vi "VTI_Split_Cluster.vi"(0 "VTI":T2={"Temperatur (K)"=0.0, "Setpoint (K)"=0.0, "Rate (K/min)"=3.4572, "Heater (%)"=0.0, "NV (%)"=0.0, "Heater Manual"=FALSE, "NV Manual"=FALSE, "Go to Set"=FALSE, "Pressure"=0.0, "Heater SP"=0.0, "Valid?"=FALSE, "Set Heater SP"=FALSE, "Set NV SP"=FALSE, "Heater (%) Display"=3.4572, "NV (%) Display"=3.4572, "NV Setpoint"=0.0, "Change Heater Status"=FALSE, "Change NV Status"=FALSE, "Sample 3"=0.0, "Sample 2"=0.0, "Sweep-State"=FALSE, "Set Auto PID"=FALSE, "Auto PID"=FALSE, "Stopp"=FALSE, "Setpoint-Sweep"=0.0} {"NV (%) Display" format="%4_5f"; "Heater (%) Display" format="%4_5f"; "Pressure" format="%#4_5f"; "NV (%)" scale=0.0..100.0; "Heater (%)" scale=0.0..100.0; "Rate (K/min)" format="%#4_5f"; "Setpoint (K)" format="%6_5f"}) -> (1 "VTI Status":T3={"Temperatur (K)"=70.6986, "Heater (%)"=0.0017142857142857142, "NV (%)"=0.0, "Heater Manual"=TRUE, "NV Manual"=TRUE, "Pressure"=1.0208606, "Valid?"=FALSE, "Heater (%) Display"=0.0, "NV (%) Display"=0.0, "Sample 2"=70.6986, "Sample 3"=70.6986, "Auto PID"=TRUE, "Sweep-Status"=TRUE, "Setpoint-Sweep"=70.6986} {"Heater (%)" scale=0.0..100.0; "NV (%)" scale=0.0..100.0}, 2 "VTI Control":T1)   [LabVIEW 2016]
uses:
  S16/VTI-status.ctl
  S16/VTI-cluster.ctl
  S16/VTI-control.ctl
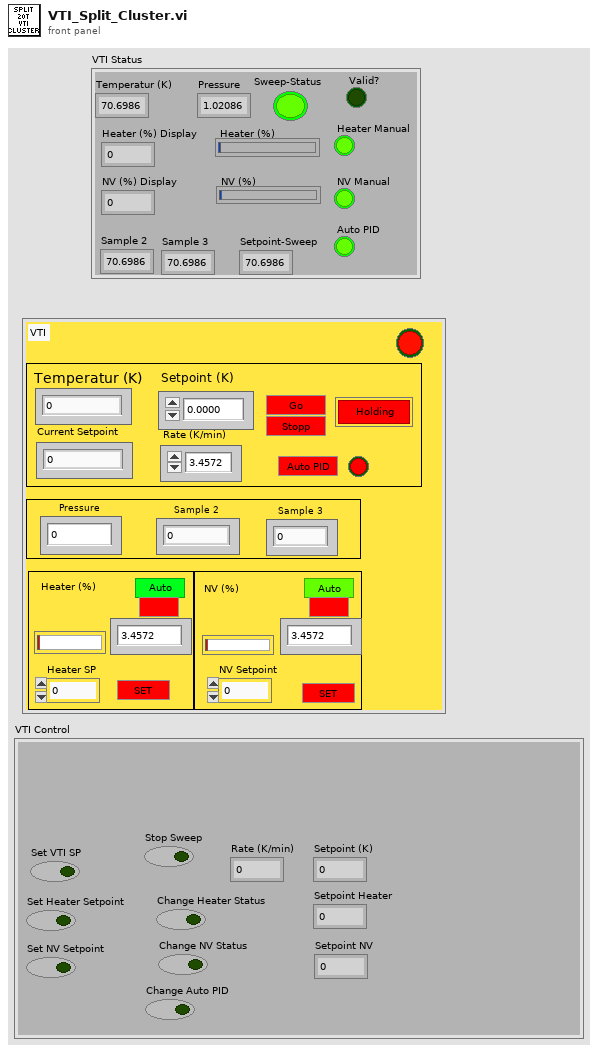
[diagram p1: front panel]
types:
  T1 = typedef "VTI-control.ctl" = cluster{"Set VTI SP":bool, "Change NV Status":bool, "Set NV Setpoint":bool, "Change Heater Status":bool, "Set Heater Setpoint":bool, "Setpoint (K)":dbl, "Rate (K/min)":dbl, "Setpoint Heater":dbl, "Setpoint NV":dbl, "Change Auto PID":bool, "Stop Sweep":bool}
  T2 = typedef "VTI-cluster.ctl" = cluster{"Temperatur (K)":dbl, "Setpoint (K)":dbl, "Rate (K/min)":dbl, "Heater (%)":dbl, "NV (%)":dbl, "Heater Manual":bool, "NV Manual":bool, "Go to Set":bool, "Pressure":dbl, "Heater SP":dbl, "Valid?":bool, "Set Heater SP":bool, "Set NV SP":bool, "Heater (%) Display":dbl, "NV (%) Display":dbl, "NV Setpoint":dbl, "Change Heater Status":bool, "Change NV Status":bool, "Sample 3":dbl, "Sample 2":dbl, "Sweep-State":bool, "Set Auto PID":bool, "Auto PID":bool, "Stopp":bool, "Setpoint-Sweep":dbl}
  T3 = typedef "VTI-status.ctl" = cluster{"Temperatur (K)":dbl, "Heater (%)":dbl, "NV (%)":dbl, "Heater Manual":bool, "NV Manual":bool, "Pressure":dbl, "Valid?":bool, "Heater (%) Display":dbl, "NV (%) Display":dbl, "Sample 2":dbl, "Sample 3":dbl, "Auto PID":bool, "Sweep-Status":bool, "Setpoint-Sweep":dbl}
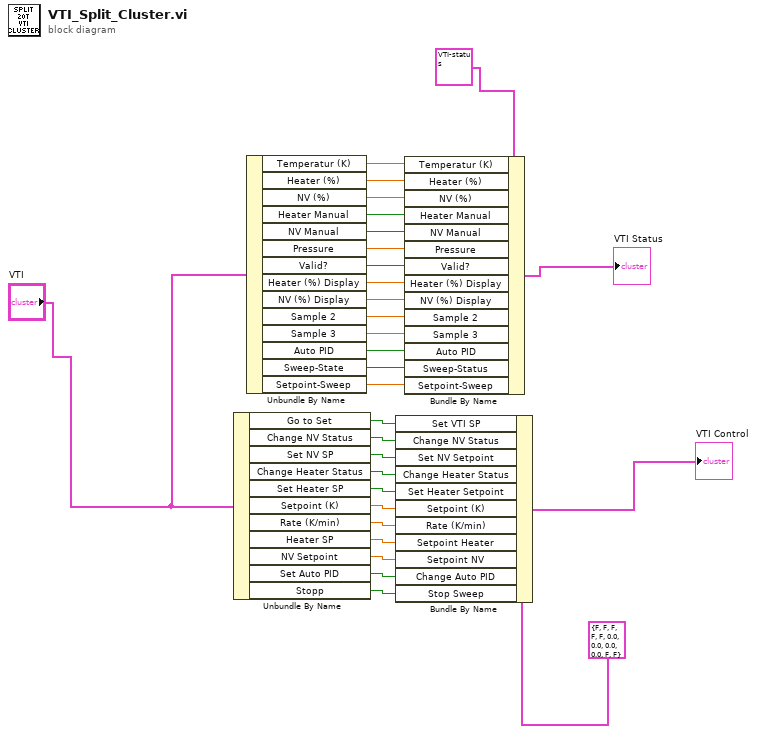
[diagram p0: block diagram]
diagram:
  n1 = Unbundle By Name("VTI") -> ("Go to Set"=w30:bool, "Change NV Status"=w29:bool, "Set NV SP"=w28:bool, "Change Heater Status"=w18:bool, "Set Heater SP"=w19:bool, "Setpoint (K)"=w20:dbl, "Rate (K/min)"=w21:dbl, "Heater SP"=w22:dbl, "NV Setpoint"=w23:dbl, "Set Auto PID"=w4:bool, "Stopp"=w2:bool)
  n2 = Unbundle By Name("VTI") -> ("Temperatur (K)"=w16:dbl, "Heater (%)"=w15:dbl, "NV (%)"=w14:dbl, "Heater Manual"=w13:bool, "NV Manual"=w12:bool, "Pressure"=w11:dbl, "Valid?"=w10:bool, "Heater (%) Display"=w9:dbl, "NV (%) Display"=w8:dbl, "Sample 2"=w7:dbl, "Sample 3"=w6:dbl, "Auto PID"=w5:bool, "Sweep-State"=w3:bool, "Setpoint-Sweep"=w1:dbl)
  n3 = Bundle By Name(cluster=T1 {"Set VTI SP"=FALSE, "Change NV Status"=FALSE, "Set NV Setpoint"=FALSE, "Change Heater Status"=FALSE, "Set Heater Setpoint"=FALSE, "Setpoint (K)"=0.0, "Rate (K/min)"=0.0, "Setpoint Heater"=0.0, "Setpoint NV"=0.0, "Change Auto PID"=FALSE, "Stop Sweep"=FALSE} ("VTI Control"), "Set VTI SP"=w30, "Change NV Status"=w29, "Set NV Setpoint"=w28, "Change Heater Status"=w18, "Set Heater Setpoint"=w19, "Setpoint (K)"=w20, "Rate (K/min)"=w21, "Setpoint Heater"=w22, "Setpoint NV"=w23, "Change Auto PID"=w4, "Stop Sweep"=w2) -> (→"VTI Control":T1)
  n4 = Bundle By Name(cluster=T3 {"Temperatur (K)"=70.6986, "Heater (%)"=0.0017142857142857142, "NV (%)"=0.0, "Heater Manual"=TRUE, "NV Manual"=TRUE, "Pressure"=1.0208606, "Valid?"=FALSE, "Heater (%) Display"=0.0, "NV (%) Display"=0.0, "Sample 2"=70.6986, "Sample 3"=70.6986, "Auto PID"=TRUE, "Sweep-Status"=TRUE, "Setpoint-Sweep"=70.6986} ("VTI Status"), "Temperatur (K)"=w16, "Heater (%)"=w15, "NV (%)"=w14, "Heater Manual"=w13, "NV Manual"=w12, "Pressure"=w11, "Valid?"=w10, "Heater (%) Display"=w9, "NV (%) Display"=w8, "Sample 2"=w7, "Sample 3"=w6, "Auto PID"=w5, "Sweep-Status"=w3, "Setpoint-Sweep"=w1) -> (→"VTI Status":T3)
